vi "TRITON_TICKS_TO_TIME.vi"(1 "Initial millisecond timer value":u32) -> (0 "Elapsed Time in Seconds":dbl)   [LabVIEW 2009]
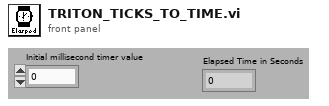
[diagram p1: front panel]
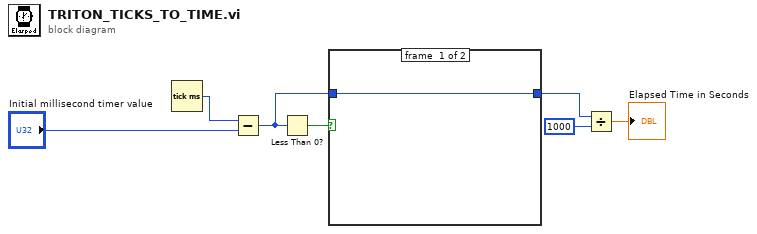
[diagram p0: block diagram]
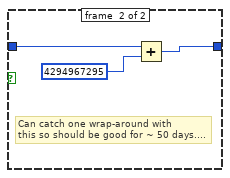
[diagram p2: hidden frame]
diagram:
  n1 = Tick Count (ms)() -> (millisecond timer value=w5:u32)
  n2 = Subtract(x=w5, y="Initial millisecond timer value") -> (x-y=w2:u32)
  n3 = Less Than 0?(x=w2) -> (x < 0?=w3:bool)
  n4 = case shown="True" w3 {
    tunnel: w2 -> [w8 w10]
    tunnel: [w8 w11] -> w1
    frame #0 {
    }
    frame #1 {
      # "Can catch one wrap-around with\nthis so should be good for ~ 50 days...."
      n5 = Add(x=w10, y=u32 4294967295) -> (x+y=w11:u32)
    }
  }
  n6 = Divide(x=w1, y=u32 1000) -> (x/y=→"Elapsed Time in Seconds":dbl)
